vi "Begin.vi"(8 "error in":errorcluster) -> (0 "error out":errorcluster)   [LabVIEW 2020]
doc: "Called before other user functions, this VI is expected to open initial I/O refnums, load in file data, and do all program initialization. Notice that the <B>error out</B> terminal is simply used for data flow. Wiring it to other structures or subVIs ensures that this VI runs first."
uses:
  <vilib>/Rock Robotics/WPI/DriverStation/WPI_DriverStationRobotMode2.ctl
  <vilib>/Rock Robotics/WPI/Joystick/WPI_JoystickDeviceEnum.ctl
  <vilib>/Rock Robotics/WPI/ThirdParty/Phoenix-LabVIEW/Motor Controller/Controls/CTRE_Phoenix_MotorControl_FeedbackDevice_TalonFX.ctl
  <vilib>/Rock Robotics/WPI/SafetyOutput/WPI_SafetyOutputConfigMenu.ctl
  <vilib>/Rock Robotics/WPI/RobotDrive/WPI_RobotDriveDevRef.ctl
  <vilib>/Rock Robotics/WPI/MotorControl/WPI_MotorControlDeviceRef.ctl
  <vilib>/Rock Robotics/WPI/MotorControl/WPI_MotorControlType.ctl
  <vilib>/Rock Robotics/SystemInterfaces/DIO/FPGA_DIOPWMChannel.ctl
  <vilib>/Rock Robotics/WPI/PWM/WPI_PWMDeadband.ctl
  <vilib>/Rock Robotics/SystemInterfaces/DIO/FPGA_DIOChannel.ctl
  <vilib>/Rock Robotics/WPI/Solenoid/WPI_SolenoidChannel.ctl
  Robot Global Data.vi
  <vilib>/Rock Robotics/Network Tables/NT Write String Array.vi
  <vilib>/Rock Robotics/WPI/Utilities/WPI_GetSetVariantRefNum.vi
  <vilib>/Rock Robotics/WPI/Solenoid/WPI_SolenoidOpenDouble.vi
  <vilib>/Rock Robotics/WPI/ThirdParty/Phoenix-LabVIEW/Pigeon IMU/CTRE_PigeonIMU_Open_CAN.vi
  <vilib>/Rock Robotics/Network Tables/NT Write Number.vi
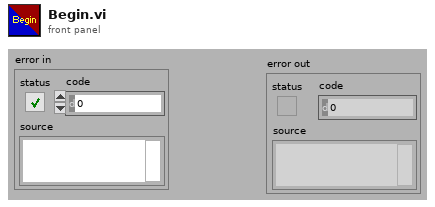
[diagram p1: front panel]
types:
  T1 = typedef "FPGA_DIOChannel.ctl" = enum8{"DIO 0", "DIO 1", "DIO 2", "DIO 3", "DIO 4", "DIO 5", "DIO 6", "DIO 7", "DIO 8", "DIO 9", "DIO MXP 0", "DIO MXP 1", "DIO MXP 2", "DIO MXP 3", "DIO MXP 4", "DIO MXP 5", "DIO MXP 6", "DIO MXP 7", "DIO MXP 8", "DIO MXP 9", "DIO MXP 10", "DIO MXP 11", "DIO MXP 12", "DIO MXP 13", "DIO MXP 14", "DIO MXP 15", "SPI Port CS1", "SPI Port CS2", "SPI Port CS3", "SPI Port MISO", "SPI Port MOSI", "Invalid"}
  T2 = typedef "WPI_SolenoidChannel.ctl" = enum8{"Solenoid 0", "Solenoid 1", "Solenoid 2", "Solenoid 3", "Solenoid 4", "Solenoid 5", "Solenoid 6", "Solenoid 7", "Solenoid 8", "Solenoid 9", "Solenoid 10", "Solenoid 11", "Solenoid 12", "Solenoid 13", "Solenoid 14", "Solenoid 15", "Invalid"}
  T3 = typedef "WPI_RobotDriveDevRef.ctl" = cluster{"DevStatus":errorcluster, "Motors[]":T4[], "Square Inputs":bool, "Max Output":dbl}
  T4 = typedef "WPI_MotorControlDeviceRef.ctl" = cluster{"DeviceStatus":errorcluster, "Type":T5, "PWM":cluster{"PWM Channel":T6, "DeadBand":T7}, "CAN":cluster{"Device Number":u8, "SetOutput VI Ref":variant, "GetOutput VI Ref":variant, "Enable VI Ref":variant, "Disable VI Ref":variant, "Data":variant}, "Invert":bool, "DIO PWM":cluster{"PWM \"Enable\" Channel":T6, "DIOChannel":T1, "PWM Rate":dbl}}
  T5 = typedef "WPI_MotorControlType.ctl" = enum16{"PWM", "CAN", "DIO PWM"}
  T6 = typedef "FPGA_DIOPWMChannel.ctl" = enum8{"PWM 0", "PWM 1", "PWM 2", "PWM 3", "PWM 4", "PWM 5", "PWM 6", "PWM 7", "PWM 8", "PWM 9", "PWM MXP 0", "PWM MXP 1", "PWM MXP 2", "PWM MXP 3", "PWM MXP 4", "PWM MXP 5", "PWM MXP 6", "PWM MXP 7", "PWM MXP 8", "PWM MXP 9", "Invalid"}
  T7 = typedef "WPI_PWMDeadband.ctl" = cluster{"Name":string, "maxPositivePwm":i32, "minPositivePwm":i32, "centerPwm":i32, "maxNegativePwm":i32, "minNegativePwm":i32, "angularRange":u16}
  T8 = typedef "WPI_SafetyOutputConfigMenu.ctl" = enum16{"Enable", "Disable"}
  T9 = typedef "CTRE_Phoenix_MotorControl_FeedbackDevice_TalonFX.ctl" = i8
  T10 = typedef "WPI_JoystickDeviceEnum.ctl" = enum16{"USB 0", "USB 1", "USB 2", "USB 3", "USB 4", "USB 5"}
  T11 = typedef "WPI_DriverStationRobotMode2.ctl" = enum16{"Autonomous Disabled", "Autonomous Enabled", "Teleop Disabled", "Teleop Enabled", "Disconnected", "Finish", "Test Disabled", "Test Enabled", "Emergency Stopped"}
  T12 = typedef "WPI_JoystickDevRef.ctl" = cluster{"Device":T10}
  T13 = typedef "CTRE_PigeonIMU_DeviceRef.ctl" = cluster{"DeviceStatus":errorcluster, "Device Number":u8, "Type":T14, "Device ID":u32, "Handle":u64, "UsageFrame":u32, "Library Path":path}
  T14 = typedef "CTRE_PigeonIMU_ConnectionType.ctl" = u32
  T15 = typedef "WPI_CompressorDevRef.ctl" = cluster{"DevStatus":errorcluster, "Pneumatics Control Module":u8}
  T16 = typedef "WPI_SolenoidDevRef.ctl" = cluster{"DevStatus":errorcluster, "Pneumatics Control Module":u8, "Forward Solenoid Channel":T2, "Reverse Solenoid Channel":T2}
  T17 = typedef "WPI_DigitalInputDevRef.ctl" = cluster{"DevStatus":errorcluster, "DIO Channel":T1}
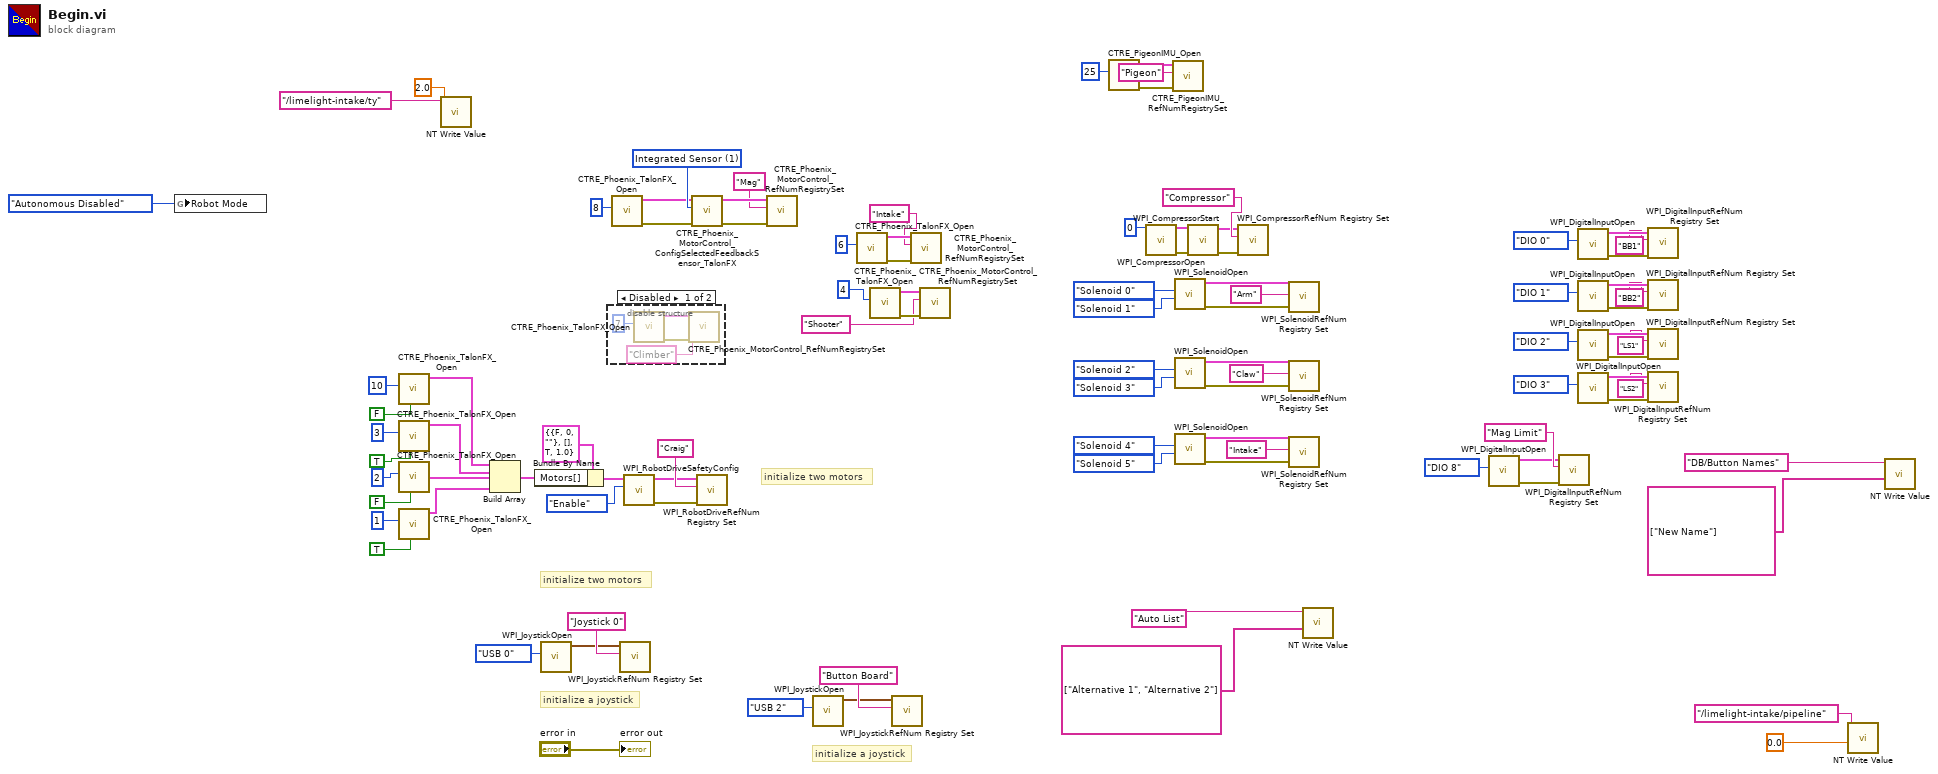
[diagram p0: block diagram]
diagram:
  w73 = T9 1 items=["Integrated Sensor"=1, "Sensor Sum (S0 + S1)"=9, "Sensor Difference (D0 - D1)"=10, "Remote Source 0"=11, "Remote Source 1"=12, "None"=14, "Software Emulated"=15] ("Talon FX Feedback Device")
  # "initialize a joystick"
  # "initialize two motors"
  # "initialize a joystick"
  # "initialize two motors"
  n1 = global write "Robot Global Data.vi" "Robot Mode"(WPI_DriverStationRobotMode2."Autonomous Disabled" ("Robot Mode")) -> ()
  n2 = call <vilib>:"CTRE_Phoenix_TalonFX_Open.vi"("Invert"=FALSE, "Device Number"=u8 10) -> ("PhoenixMotorControlDevRef"=w52:T4)  [unwired: 8 in, 1 out]
  n3 = call <vilib>:"CTRE_Phoenix_TalonFX_Open.vi"("Invert"=TRUE, "Device Number"=u8 3) -> ("PhoenixMotorControlDevRef"=w60:T4)  [unwired: 8 in, 1 out]
  n4 = call <vilib>:"CTRE_Phoenix_TalonFX_Open.vi"("Invert"=FALSE, "Device Number"=u8 2) -> ("PhoenixMotorControlDevRef"=w61:T4)  [unwired: 8 in, 1 out]
  n5 = call <vilib>:"CTRE_Phoenix_TalonFX_Open.vi"("Invert"=TRUE, "Device Number"=u8 1) -> ("PhoenixMotorControlDevRef"=w62:T4)  [unwired: 8 in, 1 out]
  n6 = call-poly <vilib>:"NT Write Value.vi"("Numeric"=2.0, "Name"="/limelight-intake/ty") -> ()  [unwired: 9 in, 1 out]
  n7 = Build Array(w52, w60, w61, w62) -> (w63:T4[])
  n8 = Bundle By Name(cluster=T3 {"DevStatus"={"status"=FALSE, "code"=0, "source"=""}, "Motors[]"=[], "Square Inputs"=TRUE, "Max Output"=1.0} ("RobotDriveDevRef"), "Motors[]"=w63) -> (w57:T3)
  n9 = call <vilib>:"WPI_JoystickOpen.vi"("JoystickDevice"=WPI_JoystickDeviceEnum."USB 0") -> ("JoystickDevRef"=w93:T12)  [unwired: 10 in]
  n10 = disable-structure shown="Disabled" {
    frame Disabled {
      n11 = call <vilib>:"CTRE_Phoenix_TalonFX_Open.vi"("Device Number"=u8 7) -> ("error out"=w99:errorcluster, "PhoenixMotorControlDevRef"=w98:T4)  [unwired: 9 in]
      n12 = call <vilib>:"CTRE_Phoenix_MotorControl_RefNumRegistrySet.vi"("error in (no error)"=w99, "refnum name"="Climber", "PhoenixMotorControlDevRef"=w98) -> ()  [unwired: 7 in, 2 out]
    }
    frame Enabled {
    }
  }
  n13 = call <vilib>:"CTRE_Phoenix_TalonFX_Open.vi"("Device Number"=u8 8) -> ("error out"=w9:errorcluster, "PhoenixMotorControlDevRef"=w10:T4)  [unwired: 9 in]
  n14 = call <vilib>:"WPI_JoystickRefNum Registry Set.vi"("refnum name"="Joystick 0", "JoystickDevRef"=w93) -> ()  [unwired: 8 in, 2 out]
  n15 = call <vilib>:"WPI_RobotDriveSafetyConfig.vi"("mode"=WPI_SafetyOutputConfigMenu."Enable", "RobotDriveDevRef"=w57) -> ("error out"=w65:errorcluster, "RobotDriveDevRef"=w64:T3)  [unwired: 2 in, 6 out]
  n16 = call <vilib>:"CTRE_Phoenix_MotorControl_ConfigSelectedFeedbackSensor_TalonFX.vi"("error in (no error)"=w9, "Talon FX Feedback Device"=w73, "PhoenixMotorControlDevRef"=w10) -> ("error out"=w74:errorcluster, "PhoenixMotorControlDevRef"=w75:T4)  [unwired: 7 in]
  n17 = call <vilib>:"WPI_RobotDriveRefNum Registry Set.vi"("error in (no error)"=w65, "refnum name"="Craig", "RobotDriveDevRef"=w64) -> ()  [unwired: 7 in, 2 out]
  n18 = call <vilib>:"CTRE_Phoenix_MotorControl_RefNumRegistrySet.vi"("error in (no error)"=w74, "refnum name"="Mag", "PhoenixMotorControlDevRef"=w75) -> ()  [unwired: 7 in, 2 out]
  n19 = call <vilib>:"WPI_JoystickOpen.vi"("JoystickDevice"=WPI_JoystickDeviceEnum."USB 2") -> ("JoystickDevRef"=w85:T12)  [unwired: 10 in]
  n20 = call <vilib>:"CTRE_Phoenix_TalonFX_Open.vi"("Device Number"=u8 6) -> ("error out"=w80:errorcluster, "PhoenixMotorControlDevRef"=w83:T4)  [unwired: 9 in]
  n21 = call <vilib>:"CTRE_Phoenix_TalonFX_Open.vi"("Device Number"=u8 4) -> ("error out"=w78:errorcluster, "PhoenixMotorControlDevRef"=w79:T4)  [unwired: 9 in]
  n22 = call <vilib>:"WPI_JoystickRefNum Registry Set.vi"("refnum name"="Button Board", "JoystickDevRef"=w85) -> ()  [unwired: 8 in, 2 out]
  n23 = call <vilib>:"CTRE_Phoenix_MotorControl_RefNumRegistrySet.vi"("error in (no error)"=w80, "refnum name"="Intake", "PhoenixMotorControlDevRef"=w83) -> ()  [unwired: 7 in, 2 out]
  n24 = call <vilib>:"CTRE_Phoenix_MotorControl_RefNumRegistrySet.vi"("error in (no error)"=w78, "refnum name"="Shooter", "PhoenixMotorControlDevRef"=w79) -> ()  [unwired: 7 in, 2 out]
  n25 = call-poly <vilib>:"CTRE_PigeonIMU_Open.vi"("Device Number"=u8 25) -> ("error out"=w7:errorcluster, "PigeonIMUDevRef"=w8:T13)  [unwired: 9 in]
  n26 = call <vilib>:"WPI_CompressorOpen.vi"("Pneumatics device (def)"=u8 0) -> ("CompressorDevRef"=w18:T15, "error out"=w19:errorcluster)  [unwired: 13 in]
  n27 = call <vilib>:"CTRE_PigeonIMU_RefNumRegistrySet.vi"("error in (no error)"=w7, "refnum name"="Pigeon", "PigeonIMUDevRef"=w8) -> ()  [unwired: 7 in, 2 out]
  n28 = call-poly <vilib>:"WPI_SolenoidOpen.vi"("Reverse Solenoid Channel"=WPI_SolenoidChannel."Solenoid 1", "Forward Solenoid Channel"=WPI_SolenoidChannel."Solenoid 0" ("Solenoid Channel")) -> ("error out"=w22:errorcluster, "SolenoidDevRef"=w23:T16)  [unwired: 8 in]
  n29 = call-poly <vilib>:"WPI_SolenoidOpen.vi"("Reverse Solenoid Channel"=WPI_SolenoidChannel."Solenoid 3", "Forward Solenoid Channel"=WPI_SolenoidChannel."Solenoid 2" ("Solenoid Channel")) -> ("error out"=w27:errorcluster, "SolenoidDevRef"=w28:T16)  [unwired: 8 in]
  n30 = call-poly <vilib>:"WPI_SolenoidOpen.vi"("Reverse Solenoid Channel"=WPI_SolenoidChannel."Solenoid 5", "Forward Solenoid Channel"=WPI_SolenoidChannel."Solenoid 4" ("Solenoid Channel")) -> ("error out"=w32:errorcluster, "SolenoidDevRef"=w33:T16)  [unwired: 8 in]
  n31 = call <vilib>:"WPI_CompressorStart.vi"("error in (no error)"=w19, "CompressorDevRef"=w18) -> ("error out"=w16:errorcluster, "CompressorDevRef"=w17:T15)  [unwired: 8 in]
  n32 = call <vilib>:"WPI_CompressorRefNum Registry Set.vi"("error in (no error)"=w16, "refnum name"="Compressor", "CompressorDevRef"=w17) -> ()  [unwired: 7 in, 2 out]
  n33 = call <vilib>:"WPI_SolenoidRefNum Registry Set.vi"("error in (no error)"=w22, "refnum name"="Arm", "SolenoidDevRef"=w23) -> ()  [unwired: 7 in, 2 out]
  n34 = call <vilib>:"WPI_SolenoidRefNum Registry Set.vi"("error in (no error)"=w27, "refnum name"="Claw", "SolenoidDevRef"=w28) -> ()  [unwired: 7 in, 2 out]
  n35 = call <vilib>:"WPI_SolenoidRefNum Registry Set.vi"("error in (no error)"=w32, "refnum name"="Intake", "SolenoidDevRef"=w33) -> ()  [unwired: 7 in, 2 out]
  n36 = call-poly <vilib>:"NT Write Value.vi"("String Array"=string[] ["Alternative 1", "Alternative 2"], "Name"="Auto List") -> ()  [unwired: 9 in, 1 out]
  n37 = call <vilib>:"WPI_DigitalInputOpen.vi"("DIO Channel"=FPGA_DIOChannel."DIO 8") -> ("error out"=w12:errorcluster, "DigitalInputDevRef"=w13:T17)  [unwired: 9 in]
  n38 = call <vilib>:"WPI_DigitalInputRefNum Registry Set.vi"("error in (no error)"=w12, "refnum name"="Mag Limit", "DigitalInputDevRef"=w13) -> ()  [unwired: 7 in, 2 out]
  n39 = call <vilib>:"WPI_DigitalInputOpen.vi"("DIO Channel"=FPGA_DIOChannel."DIO 0") -> ("error out"=w41:errorcluster, "DigitalInputDevRef"=w40:T17)  [unwired: 9 in]
  n40 = call <vilib>:"WPI_DigitalInputOpen.vi"("DIO Channel"=FPGA_DIOChannel."DIO 1") -> ("error out"=w44:errorcluster, "DigitalInputDevRef"=w43:T17)  [unwired: 9 in]
  n41 = call <vilib>:"WPI_DigitalInputOpen.vi"("DIO Channel"=FPGA_DIOChannel."DIO 2") -> ("error out"=w47:errorcluster, "DigitalInputDevRef"=w46:T17)  [unwired: 9 in]
  n42 = call <vilib>:"WPI_DigitalInputOpen.vi"("DIO Channel"=FPGA_DIOChannel."DIO 3") -> ("error out"=w50:errorcluster, "DigitalInputDevRef"=w49:T17)  [unwired: 9 in]
  n43 = call <vilib>:"WPI_DigitalInputRefNum Registry Set.vi"("error in (no error)"=w41, "refnum name"="BB1", "DigitalInputDevRef"=w40) -> ()  [unwired: 7 in, 2 out]
  n44 = call <vilib>:"WPI_DigitalInputRefNum Registry Set.vi"("error in (no error)"=w44, "refnum name"="BB2", "DigitalInputDevRef"=w43) -> ()  [unwired: 7 in, 2 out]
  n45 = call <vilib>:"WPI_DigitalInputRefNum Registry Set.vi"("error in (no error)"=w47, "refnum name"="LS1", "DigitalInputDevRef"=w46) -> ()  [unwired: 7 in, 2 out]
  n46 = call <vilib>:"WPI_DigitalInputRefNum Registry Set.vi"("error in (no error)"=w50, "refnum name"="LS2", "DigitalInputDevRef"=w49) -> ()  [unwired: 7 in, 2 out]
  n47 = call-poly <vilib>:"NT Write Value.vi"("Numeric"=0.0, "Name"="/limelight-intake/pipeline") -> ()  [unwired: 9 in, 1 out]
  n48 = call-poly <vilib>:"NT Write Value.vi"("String Array"=string[] ["New Name"], "Name"="DB/Button Names") -> ()  [unwired: 9 in, 1 out]
  "error out" <- "error in"
